vi "TDMS - AeroQuad File Viewer.vi"(4 "error in (no error)":errorcluster, 7 "file path":path) -> (0 "error out":errorcluster, 3 "file path out":path)   [LabVIEW 2009]
doc: "Opens the .tdms file specified in the <B>file path</B> input and presents the file data in the TDMS File Viewer dialog box."
uses:
  <vilib>/Utility/tdmsutil.llb/fileViewerConfigData.ctl
  Instance           1 26Saved   TDMS - File Viewer .vi
  <vilib>/Utility/tdmsutil.llb/TDMSFileViewerLocalizedText.vi
  <vilib>/Utility/error.llb/DialogType.ctl
panel:
  in  "Help":bool
  in  "Status":string
  in  "Quit":bool
  in  "Settings...":bool
  in  "Properties / Values / Graph":T1(tab)
  in  "Properties":i32(listbox)
  in  "Raw data values":i32(listbox)
  out "Waveform Graph":waveform(dbl)[](graph)
  in  "File contents":string(tree)
  # "Displaying values 1..1000"
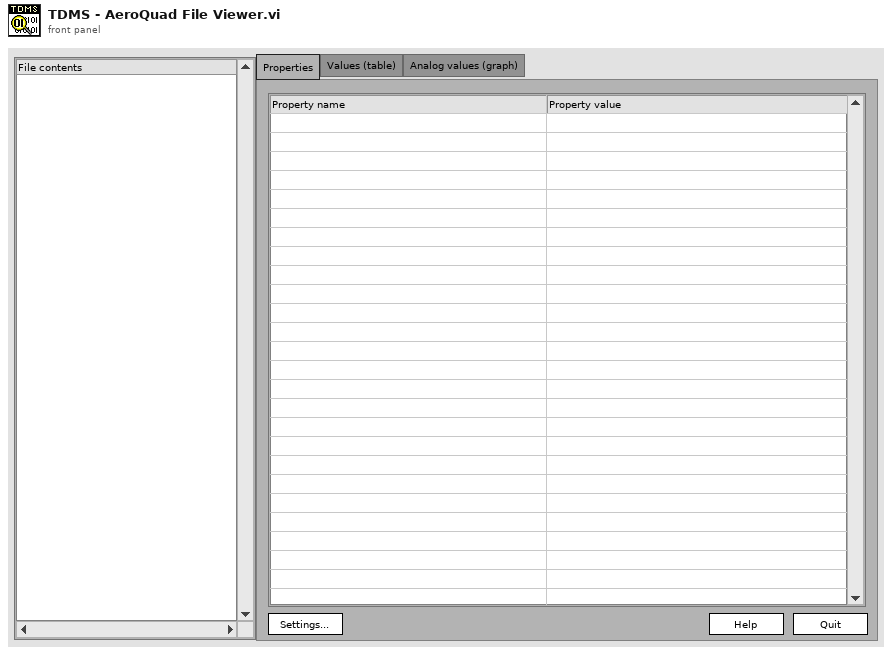
[diagram p1: front panel]
types:
  T1 = enum32{"Properties", "Values (table)", "Analog values (graph)"}
  T2 = enum16{"open", "open or create", "create or replace", "create", "open (read-only)"}
  T3 = typedef "fileViewerConfigData.ctl" = cluster{"Show all (table)":bool, "Show all (graph)":bool, "limit (table)":u64, "limit (graph)":u64, "no show":bool, "start (table)":u64, "start (graph)":u64}
  T4 = cluster{"Tree":refnum<vi>, "Tab Control":refnum<vi>, "property list":refnum<vi>, "raw data list":refnum<vi>, "Waveform Graph":refnum<vi>, "Ok":refnum<vi>, "Ok 2":refnum<vi>, "Ok 3":refnum<vi>, "Ok 4":refnum<vi>}
  T5 = typedef "LVRectTypeDef.ctl" = cluster{"left":i16, "top":i16, "right":i16, "bottom":i16}
  T6 = typedef "DialogType.ctl" = u16
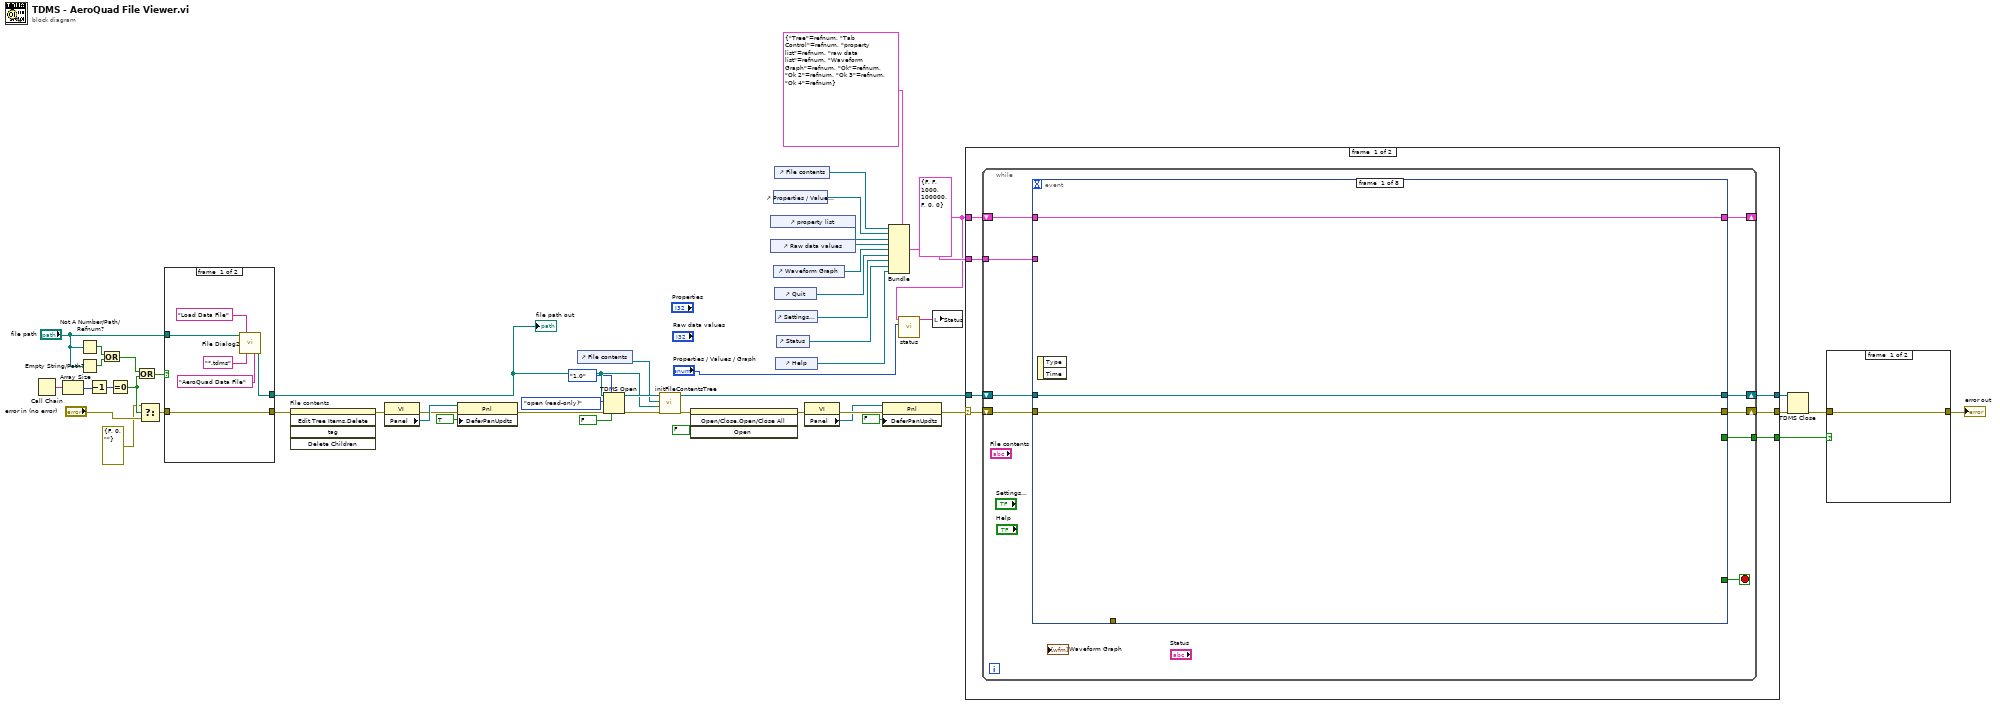
[diagram p0: block diagram]
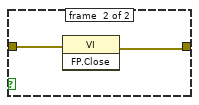
[diagram p2: hidden frame]
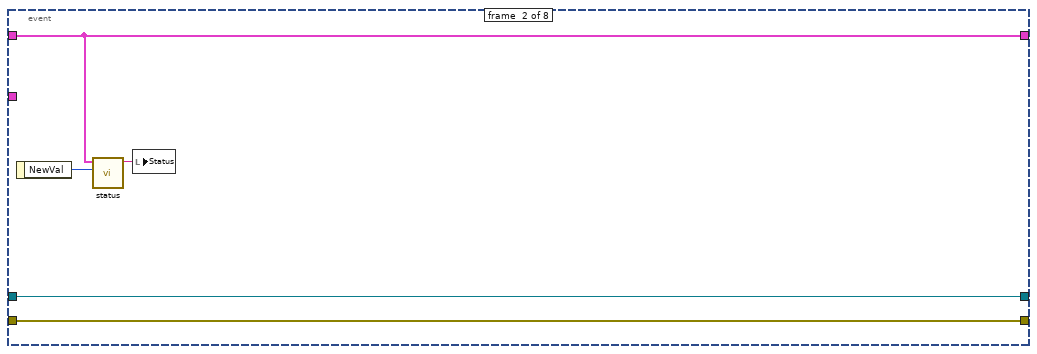
[diagram p3: hidden frame]
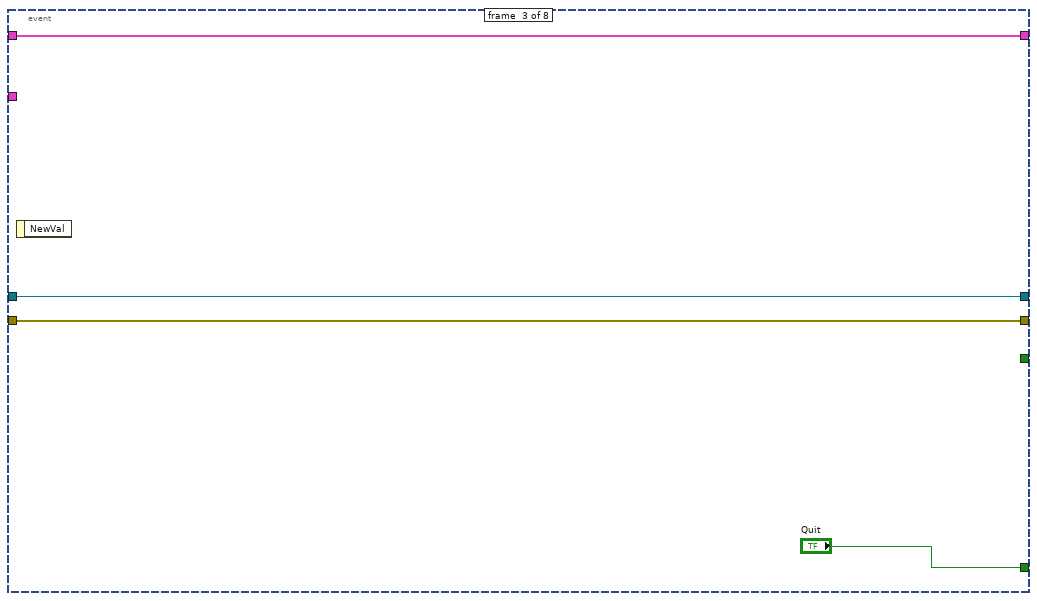
[diagram p4: hidden frame]
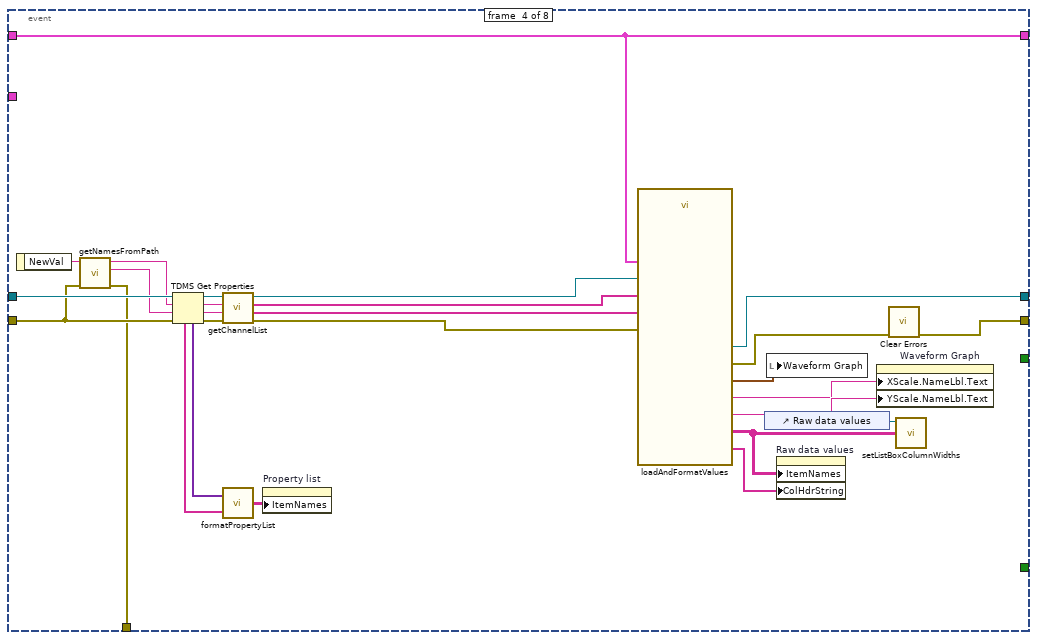
[diagram p5: hidden frame]
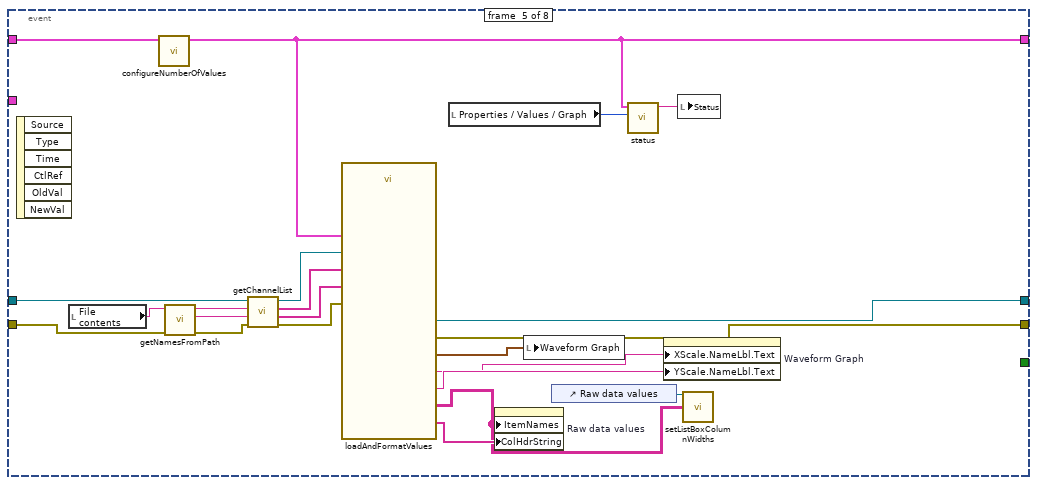
[diagram p6: hidden frame]
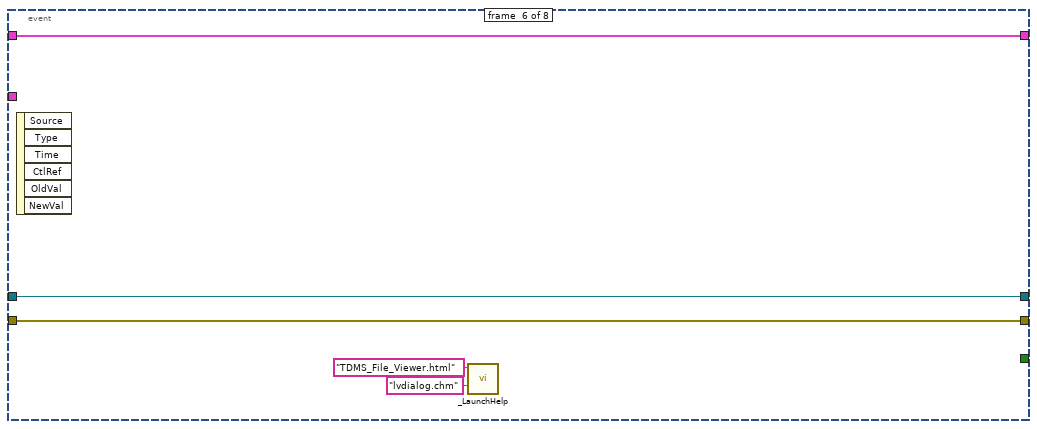
[diagram p7: hidden frame]
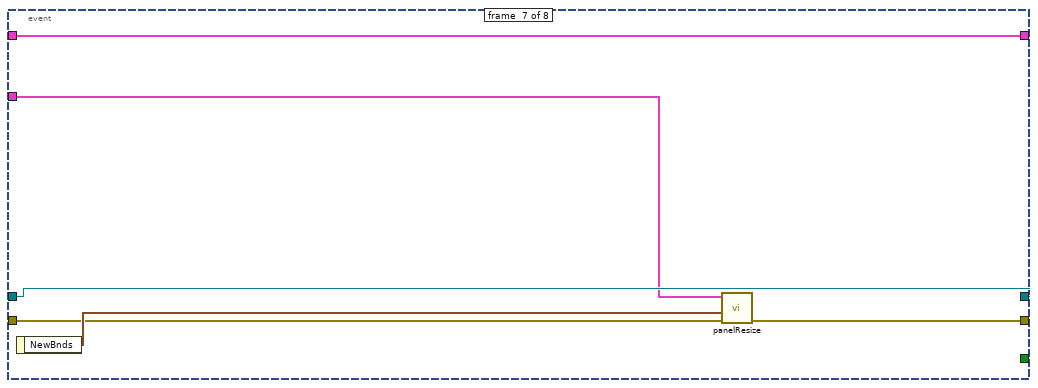
[diagram p8: hidden frame]
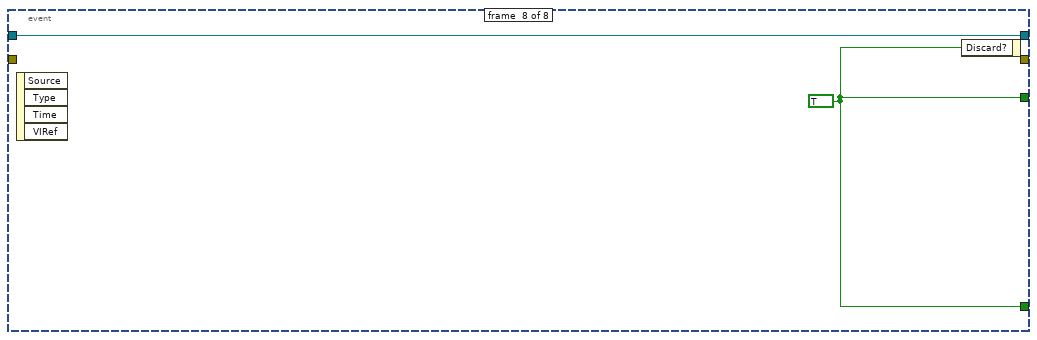
[diagram p9: hidden frame]
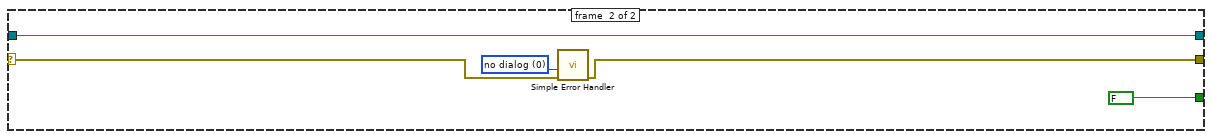
[diagram p10: hidden frame]
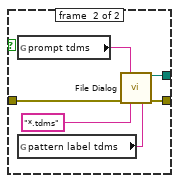
[diagram p11: hidden frame]
diagram:
  w12 = T3 {"Show all (table)"=FALSE, "Show all (graph)"=FALSE, "limit (table)"=1000, "limit (graph)"=100000, "no show"=FALSE, "start (table)"=0, "start (graph)"=0} ("TDMS File Viewer Configuration")
  n1 = Call Chain() -> (call chain=w33:string[])
  n2 = Array Size(array=w33) -> (size(s)=w31:i32)
  n3 = Not A Number/Path/Refnum?(number/path/refnum="file path") -> (NaN/Path/Refnum?=w35:bool)
  n4 = Empty String/Path?(string/path="file path") -> (empty?=w34:bool)
  n5 = Decrement(x=w31) -> (x-1=w30:i32)
  n6 = Or(x=w35, y=w34) -> (x .or. y?=w32:bool)
  n7 = Equal To 0?(x=w30) -> (x = 0?=w10:bool)
  n8 = Or(x=w32, y=w10) -> (x .or. y?=w29:bool)
  n9 = Select(t=errorcluster {"status"=FALSE, "code"=0, "source"=""}, s=w10, f="error in (no error)") -> (s? t:f=w9:errorcluster)
  n10 = case shown="False" w29 {
    tunnel: [w56 w64] -> w17
    tunnel: "file path" -> [w57 _]
    tunnel: [w58 w62] -> w16
    tunnel: w9 -> [w58 w61]
    frame #0 {
      n11 = call "File Dialog2"("start path"=w57, "prompt"="Load Data File", "pattern (all files)"="*.tdms", "pattern label"="AeroQuad Data File") -> ("selected path"=w56:path)  [unwired: 8 in, 3 out]
    }
    frame #1 {
      n12 = global read "TDMSFileViewerLocalizedText.vi" "prompt tdms"() -> (w60:string)
      n13 = global read "TDMSFileViewerLocalizedText.vi" "pattern label tdms"() -> (w59:string)
      n14 = call "File Dialog"("prompt"=w60, "error in"=w61, "pattern (all files)"="*.tdms", "pattern label"=w59) -> ("selected path"=w64:path, "error out"=w62:errorcluster)  [unwired: 3 in, 7 out]
    }
  }
  "file path out" <- w17
  n15 = invoke on="File contents" class="Tree (strict)" method="Edit Tree Items.Delete"(error in=w16) -> (error out=w43:errorcluster)  [unwired: 4 in, 4 out]
  n16 = property class="VI"(error in=w43) -> (error out=w44:errorcluster, "Panel"=w45:refnum<vi>)  [unwired: 1 in, 1 out]
  n17 = property class="Pnl"(reference=w45, error in=w44, "DeferPanUpdts"=TRUE ("Defer Panel Updates")) -> (error out=w47:errorcluster)  [unwired: 1 out]
  n18 = control-ref of="File contents"() -> (w18:refnum<vi>)
  n19 = TDMS Open(6:FALSE ("disable buffering (T)"), 7:enum16{"1.0", "2.0"}."1.0" ("file format version (2.0)"), 8:w47, 10:T2."open (read-only)" ("operation"), 11:w17) -> (0:w52:errorcluster, 3:w51:refnum<k34>)  [unwired: 1 in]
  n20 = call <vilib>:"initFileContentsTree.vi"("error in (no error)"=w52, "file path"=w17, "Tree Refnum"=w18, "tdms file"=w51) -> ("error out"=w39:errorcluster, "tdms file out"=w50:refnum<k34>)  [unwired: 2 out]
  n21 = invoke on="File contents" class="Tree (strict)" method="Open/Close.Open/Close All"(error in=w39, "Open"=FALSE ("Open?")) -> (error out=w38:errorcluster)  [unwired: 2 in, 3 out]
  n22 = control-ref of="property list"() -> (w25:refnum<vi>)
  n23 = control-ref of="Raw data values"() -> (w24:refnum<vi>)
  n24 = control-ref of="Properties / Values / Graph"() -> (w26:refnum<vi>)
  n25 = control-ref of="Waveform Graph"() -> (w23:refnum<vi>)
  n26 = control-ref of="File contents"() -> (w28:refnum<vi>)
  n27 = control-ref of="Quit"() -> (w22:refnum<vi>)
  n28 = control-ref of="Settings..."() -> (w20:refnum<vi>)
  n29 = control-ref of="Help"() -> (w1:refnum<vi>)
  n30 = control-ref of="Status"() -> (w14:refnum<vi>)
  n31 = property class="VI"(error in=w38) -> (error out=w41:errorcluster, "Panel"=w40:refnum<vi>)  [unwired: 1 in, 1 out]
  n32 = property class="Pnl"(reference=w40, error in=w41, "DeferPanUpdts"=FALSE ("Defer Panel Updates")) -> (error out=w15:errorcluster)  [unwired: 1 out]
  n33 = Bundle(cluster=T4 {"Tree"=refnum, "Tab Control"=refnum, "property list"=refnum, "raw data list"=refnum, "Waveform Graph"=refnum, "Ok"=refnum, "Ok 2"=refnum, "Ok 3"=refnum, "Ok 4"=refnum} ("control refs"), "Tree"=w28, "Tab Control"=w26, "property list"=w25, "raw data list"=w24, "Waveform Graph"=w23, "Ok"=w22, "Ok 2"=w20, "Ok 3"=w14, "Ok 4"=w1) -> (w27:T4)
  n34 = call <vilib>:"status.vi"("tab sheet"="Properties / Values / Graph", "TDMS File Viewer Configuration"=w12) -> ("status"=w13:string)  [unwired: 5 out]
  n35 = local write "Status"(w13) -> ()
  n36 = case shown="Error" w15 {
    selector: w15 -> [w66 w158]
    tunnel: w50 -> [w71 w159]
    tunnel: [w70 w159] -> w49
    tunnel: [w69 w157] -> w48
    tunnel: w27 -> [w68 _]
    tunnel: w12 -> [w67 _]
    tunnel: [w65 FALSE] -> w6
    frame #0 {
      n37 = while {
        shift-right: [w78] -> w69
        shift-left: w66 -> [w79]
        shift-right: [w77] -> w70
        shift-left: w71 -> [w80]
        tunnel: w68 -> [w75]
        shift-right: [w73] -> _
        shift-left: w67 -> [w74]
        tunnel: [w72] -> w65
        stop <- w76 stop-if-true
        n38 = event shown="[6] Panel Resize" {
          selector: _ -> [_ _ _ _ _ _ _ _]
          dyn-events: _ -> [_ _ _ _ _ _ _ _]
          timeout: _ -> [_ _ _ _ _ _ _ _]
          tunnel: w80 -> [w82 w87 w91 w119 w130 w145 w152 w154]
          tunnel: w79 -> [w83 w88 w90 w111 w138 w144 w149 _]
          tunnel: [w83 w88 w90 w106 w139 w144 w148 _] -> w78
          tunnel: [w82 w87 w91 w118 w140 w145 w152 w154] -> w77
          tunnel: [_ _ "Quit" _ _ _ _ w153] -> w76
          tunnel: [_ _ _ w110 _ _ _ _] -> _
          tunnel: w75 -> [_ _ _ _ _ _ w150 _]
          tunnel: w74 -> [w81 w84 w89 w99 w141 w146 w147 _]
          tunnel: [w81 w84 w89 w99 w120 w146 w147 _] -> w73
          tunnel: [_ _ _ _ _ _ _ w153] -> w72
          event #0 {
            n39 = event-data() -> ()  [unwired: 3 out]
          }
          event #1 {
            n40 = event-data() -> ("NewVal"=w86:T1)  [unwired: 1 out]
            n41 = call <vilib>:"status.vi"("tab sheet"=w86, "TDMS File Viewer Configuration"=w84) -> ("status"=w85:string)  [unwired: 5 out]
            n42 = local write "Status"(w85) -> ()
          }
          event #2 {
            n43 = event-data() -> ()  [unwired: 2 out]
          }
          event #3 {
            n44 = event-data() -> ("NewVal"=w113:string)  [unwired: 1 out]
            n45 = call <vilib>:"getNamesFromPath.vi"("error in (no error)"=w111, "tree path"=w113) -> ("error out"=w110:errorcluster, "channel"=w116:string, "group"=w117:string)  [unwired: 3 out]
            n46 = TDMS Get Properties(8:w111, 9:w116, 10:w117, 11:w119) -> (0:w104:errorcluster, 1:w103:string, 2:w97:string, 3:w105:refnum<k34>, 4:w114:variant[], 6:w115:string[])  [unwired: 2 out]
            n47 = call <vilib>:"getChannelList.vi"("error in (no error)"=w104, "channel names"=w103, "group name"=w97, "tdms file"=w105) -> ("error out"=w93:errorcluster, "channel names out"=w94:string[], "group names out"=w95:string[], "tdms file out"=w96:refnum<k34>)
            n48 = call <vilib>:"formatPropertyList.vi"("property names"=w115, "property values"=w114) -> ("strings"=w112:string[][])
            n49 = property on="Property list" class="MCListbox (strict)"("ItemNames"=w112) -> ()  [unwired: 2 in, 2 out]
            n50 = call <vilib>:"loadAndFormatValues.vi"("error in (no error)"=w93, "configuration"=w99, "channel names"=w94, "group names"=w95, "tdms file"=w96) -> ("error out"=w107:errorcluster, "graph y names"=w101:string, "graph x names"=w100:string, "tdms file out"=w118:refnum<k34>, "waveform values"=w98:waveform(dbl)[], "table values"=w109:string[][], "table headers"=w102:string[])
            n51 = control-ref of="Raw data values"() -> (w108:refnum<vi>)
            n52 = local write "Waveform Graph"(w98) -> ()
            n53 = property on="Raw data values" class="MCListbox (strict)"("ItemNames"=w109, "ColHdrString"=w102) -> ()  [unwired: 2 in, 2 out]
            n54 = property on="Waveform Graph" class="WFGraph (strict)"("XScale.NameLbl.Text"=w100, "YScale.NameLbl.Text"=w101) -> ()  [unwired: 2 in, 2 out]
            n55 = call <vilib>:"Clear Errors.vi"("error in (no error)"=w107) -> ("error out"=w106:errorcluster)  [unwired: 6 out]
            n56 = call <vilib>:"setListBoxColumnWidths.vi"("table data"=w109, "MCListbox Refnum"=w108) -> ()  [unwired: 1 out]
          }
          event #4 {
            n57 = event-data() -> ()  [unwired: 7 out]
            n58 = local read "File contents"() -> (w131:string)
            n59 = call <vilib>:"configureNumberOfValues.vi"("TDMS File Viewer Configuration"=w141) -> ("TDMS File Viewer Configuration Out"=w120:T3)  [unwired: 10 out]
            n60 = call <vilib>:"getNamesFromPath.vi"("error in (no error)"=w138, "tree path"=w131) -> ("error out"=w129:errorcluster, "channel"=w127:string, "group"=w128:string)  [unwired: 3 out]
            n61 = call <vilib>:"getChannelList.vi"("error in (no error)"=w129, "channel names"=w127, "group name"=w128, "tdms file"=w130) -> ("error out"=w126:errorcluster, "channel names out"=w123:string[], "group names out"=w124:string[], "tdms file out"=w125:refnum<k34>)
            n62 = call <vilib>:"loadAndFormatValues.vi"("error in (no error)"=w126, "configuration"=w120, "channel names"=w123, "group names"=w124, "tdms file"=w125) -> ("error out"=w139:errorcluster, "graph y names"=w133:string, "graph x names"=w132:string, "tdms file out"=w140:refnum<k34>, "waveform values"=w137:waveform(dbl)[], "table values"=w134:string[][], "table headers"=w136:string[])
            n63 = local read "Properties / Values / Graph"() -> (w121:T1)
            n64 = property on="Raw data values" class="MCListbox (strict)"("ItemNames"=w134, "ColHdrString"=w136) -> ()  [unwired: 2 in, 2 out]
            n65 = local write "Waveform Graph"(w137) -> ()
            n66 = control-ref of="Raw data values"() -> (w135:refnum<vi>)
            n67 = call <vilib>:"status.vi"("tab sheet"=w121, "TDMS File Viewer Configuration"=w120) -> ("status"=w122:string)  [unwired: 5 out]
            n68 = property on="Waveform Graph" class="WFGraph (strict)"("XScale.NameLbl.Text"=w132, "YScale.NameLbl.Text"=w133) -> ()  [unwired: 2 in, 2 out]
            n69 = local write "Status"(w122) -> ()
            n70 = call <vilib>:"setListBoxColumnWidths.vi"("table data"=w134, "MCListbox Refnum"=w135) -> ()  [unwired: 1 out]
          }
          event #5 {
            n71 = event-data() -> ()  [unwired: 7 out]
            n72 = call <helpdir>:"_LaunchHelp.vi"("CHM or HLP filename (lvdialog.chm)"="lvdialog.chm", "HTML filename"="TDMS_File_Viewer.html") -> ()  [unwired: 1 in, 5 out]
          }
          event #6 {
            n73 = event-data() -> ("NewBnds"=w151:T5)  [unwired: 1 out]
            n74 = call <vilib>:"panelResize.vi"("error in (no error)"=w149, "NewBnds"=w151, "control refs"=w150) -> ("error out"=w148:errorcluster)  [unwired: 4 out]
          }
          event #7 {
            w153 = TRUE
            n75 = event-data() -> ()  [unwired: 5 out]
            n76 = event-data("Discard?"=w153) -> ()  [unwired: 1 in, 1 out]
          }
        }
      }
    }
    frame #1 {
      w155 = T6 0 items=["no dialog", "OK message", "continue or stop message", "OK message + warnings", "continue/stop + warnings"] ("type of dialog (OK msg:1)")
      n77 = call <vilib>:"Simple Error Handler.vi"("type of dialog (OK msg:1)"=w155, "error in (no error)"=w158) -> ("error out"=w157:errorcluster)  [unwired: 7 out]
    }
  }
  n78 = TDMS Close(8:w48, 11:w49) -> (0:w5:errorcluster)
  n79 = case shown="True" w6 {
    tunnel: w5 -> [w160 w162]
    tunnel: [w160 w161] -> w4
    frame #0 {
    }
    frame #1 {
      n80 = invoke class="VI" method="FP.Close"(error in=w162) -> (error out=w161:errorcluster)  [unwired: 2 in, 2 out]
    }
  }
  "error out" <- w4
